vi "Create Reader Endpoint.vi"(8 "error in (no error)":errorcluster, 9 "writer name":string, 10 "reader name":string="writer", 11 "Stream in":refnum<class "Stream.lvclass">) -> (0 "error out":errorcluster, 3 "Stream out":refnum<class "Stream.lvclass">)   [LabVIEW 2018, in "Stream.lvclass"]
uses:
  Stream.lvclass
  Stream.lvclass/Stream.ctl
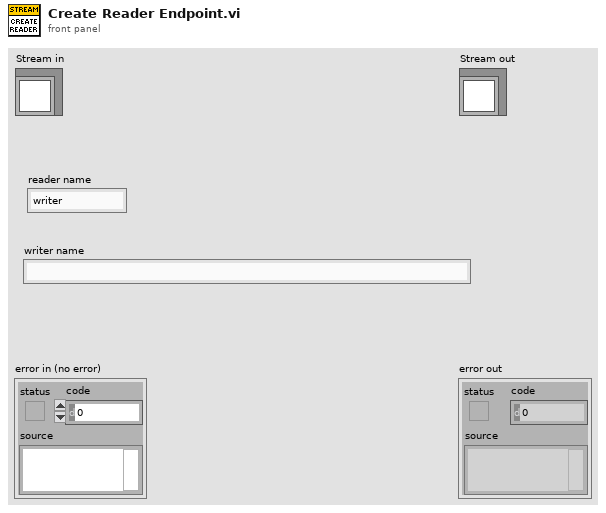
[diagram p1: front panel]
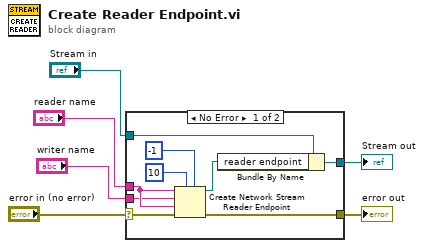
[diagram p0: block diagram]
diagram:
  n1 = case shown="No Error" "error in (no error)" {
    selector: "error in (no error)" -> [w14 w17]
    tunnel: [w15 w17] -> w4
    tunnel: [w11 w16] -> w3
    tunnel: "Stream in" -> [w12 w16]
    tunnel: "reader name" -> [w9 _]
    tunnel: "writer name" -> [w7 _]
    frame No Error {
      n2 = Create Network Stream Reader Endpoint(5:-1 ("timeout in ms (-1)"), 7:10 ("writer buffer size"), 8:w14, 9:w9, 10:w7, 11:w9) -> (0:w15:errorcluster, 3:w8:refnum<k21>)  [unwired: 1 in]
      n3 = Bundle By Name(cluster=w12, "reader endpoint"=w8) -> (w11:refnum<class "Stream.lvclass">)
    }
    frame Error {
    }
  }
  "error out" <- w4
  "Stream out" <- w3
